vi "StrDisplay.vi"(6 "Payload":u8[](array[numeric]) format="%.0x", 7 "Err str":string, 9 "ID":i32, 10 "string in":string, 11 "string type":string) -> (3 "str out":string)   [LabVIEW 2017]
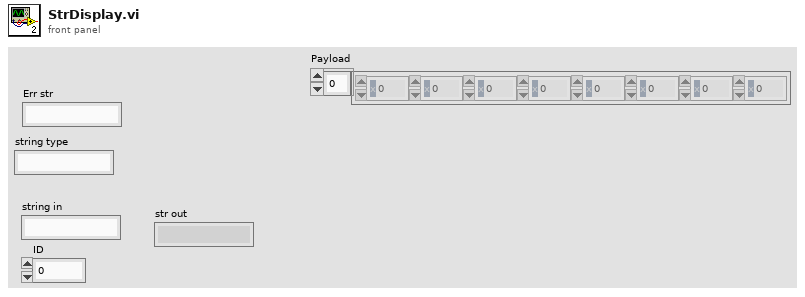
[diagram p1: front panel]
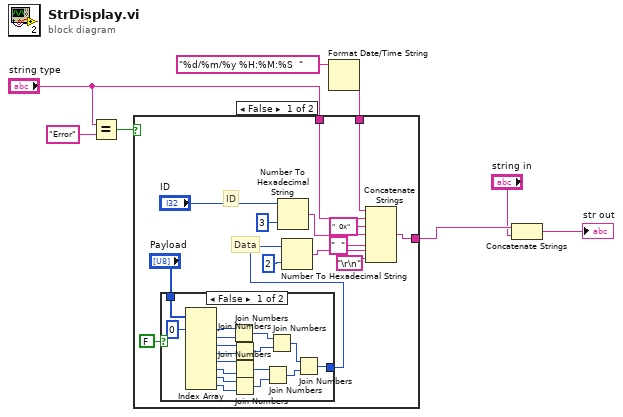
[diagram p0: block diagram]
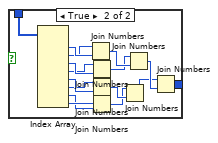
[diagram p2: hidden frame]
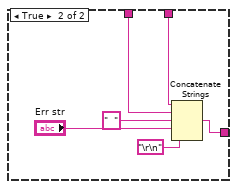
[diagram p3: hidden frame]
diagram:
  n1 = Equal?(x="string type", y="Error") -> (x = y?=w3:bool)
  n2 = Format Date/Time String(time format string (%c)="%d/%m/%y %H:%M:%S  ") -> (date/time string=w8:string)  [unwired: 2 in]
  n3 = case shown="False" w3 {
    tunnel: w8 -> [w18 w60]
    tunnel: [w16 w61] -> w6
    tunnel: "string type" -> [w15 w59]
    frame False {
      # "Data"
      # "ID"
      n4 = case shown="False" FALSE {
        tunnel: "Payload" -> [w39 w55]
        tunnel: [w23 w40] -> w10
        frame False {
          n5 = Index Array(array=w39, index #1=0 ("index")) -> (element #1=w37:u8, element #2=w36:u8, element #3=w35:u8, element #4=w34:u8, element #5=w33:u8, element #6=w32:u8, element #7=w31:u8, element #8=w30:u8)  [unwired: 7 in]
          n6 = Join Numbers(hi=w37, lo=w36) -> ((hi.lo)=w29:u16)
          n7 = Join Numbers(hi=w35, lo=w34) -> ((hi.lo)=w28:u16)
          n8 = Join Numbers(hi=w33, lo=w32) -> ((hi.lo)=w27:u16)
          n9 = Join Numbers(hi=w31, lo=w30) -> ((hi.lo)=w26:u16)
          n10 = Join Numbers(hi=w27, lo=w26) -> ((hi.lo)=w24:u32)
          n11 = Join Numbers(hi=w29, lo=w28) -> ((hi.lo)=w25:u32)
          n12 = Join Numbers(hi=w25, lo=w24) -> ((hi.lo)=w23:u64)
        }
        frame True {
          n13 = Index Array(array=w55) -> (element #1=w54:u8, element #2=w53:u8, element #3=w52:u8, element #4=w51:u8, element #5=w48:u8, element #6=w47:u8, element #7=w45:u8, element #8=w46:u8)  [unwired: 8 in]
          n14 = Join Numbers(hi=w53, lo=w54) -> ((hi.lo)=w50:u16)
          n15 = Join Numbers(hi=w51, lo=w52) -> ((hi.lo)=w49:u16)
          n16 = Join Numbers(hi=w47, lo=w48) -> ((hi.lo)=w44:u16)
          n17 = Join Numbers(hi=w46, lo=w45) -> ((hi.lo)=w43:u16)
          n18 = Join Numbers(hi=w43, lo=w44) -> ((hi.lo)=w41:u32)
          n19 = Join Numbers(hi=w49, lo=w50) -> ((hi.lo)=w42:u32)
          n20 = Join Numbers(hi=w41, lo=w42) -> ((hi.lo)=w40:u64)
        }
      }
      n21 = Number To Hexadecimal String(1:i16 3 ("width (-)"), 2:"ID") -> (0:w20:string)
      n22 = Number To Hexadecimal String(1:i16 2 ("width (-)"), 2:w10) -> (0:w22:string)
      n23 = Concatenate Strings(w18, w15, "  0x" ("string"), w20, "  " ("string"), w22, "\r\n") -> (w16:string)
    }
    frame True {
      n24 = Concatenate Strings(w60, w59, "  " ("string"), "Err str", "\r\n") -> (w61:string)
    }
  }
  n25 = Concatenate Strings(w6, "string in") -> (→"str out":string)
